vi "Selection.Convert.Set.vi"(8 "error in (no error)":errorcluster, 10 "Selections":T1={"Pull In Time"=FALSE, "Pull In Max Current"=FALSE, "Pull In Max Voltage"=TRUE, "Pull In Min Voltage"=TRUE, "Pull In Avg Voltage"=FALSE, "Hold Time"=FALSE, "Hold Max Current"=FALSE, "Hold Min Current"=FALSE, "Hold Avg Current"=FALSE, "Hold Max Voltage"=FALSE, "Hold Min Voltage"=FALSE, "Hold Avg Max Voltage"=FALSE, "Hold Avg Min Voltage"=FALSE, "Off Time"=FALSE, "Off Max Current"=FALSE, "Off Min Current"=FALSE, "Off Avg Current"=FALSE, "Off Max Voltage"=FALSE, "Off Min Voltage"=TRUE, "Off Avg Voltage"=FALSE, "Total Voltage Pulses"=FALSE, "Total Stage Time"=TRUE}, 11 "ListBox in":refnum<vi>) -> (0 "error out":errorcluster)   [LabVIEW 2019, in "Fuel Injector Analysis Addon System Explorer.lvlib"]
uses:
  Fuel Injector Analysis Addon System Explorer.lvlib
  Addon Shared/Types/Analysis.Channels.Select.ctl
  Addon Shared/Fuel Injector Analysis Addon Shared.lvlib
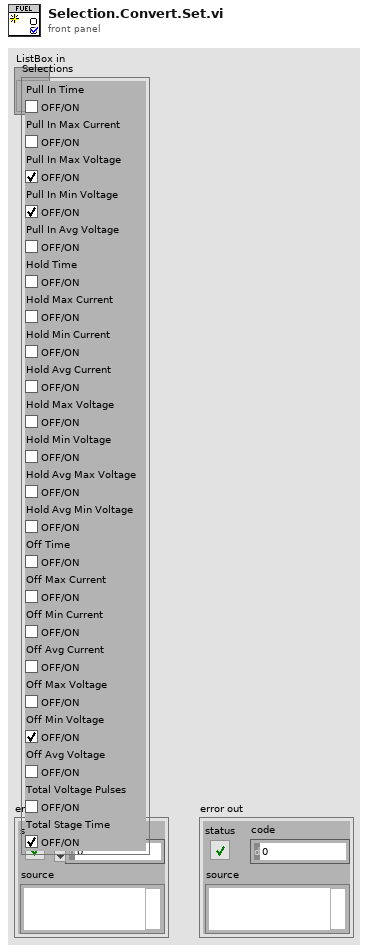
[diagram p1: front panel]
types:
  T1 = typedef "Fuel Injector Analysis Addon Shared.lvlib/Analysis.Channels.Select.ctl" = cluster{"Pull In Time":bool, "Pull In Max Current":bool, "Pull In Max Voltage":bool, "Pull In Min Voltage":bool, "Pull In Avg Voltage":bool, "Hold Time":bool, "Hold Max Current":bool, "Hold Min Current":bool, "Hold Avg Current":bool, "Hold Max Voltage":bool, "Hold Min Voltage":bool, "Hold Avg Max Voltage":bool, "Hold Avg Min Voltage":bool, "Off Time":bool, "Off Max Current":bool, "Off Min Current":bool, "Off Avg Current":bool, "Off Max Voltage":bool, "Off Min Voltage":bool, "Off Avg Voltage":bool, "Total Voltage Pulses":bool, "Total Stage Time":bool}
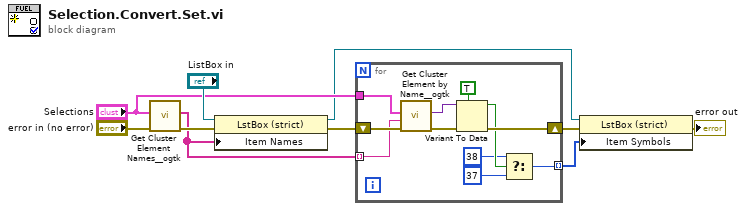
[diagram p0: block diagram]
diagram:
  n1 = call <userlib>:"Get Cluster Element Names__ogtk.vi"("error in (no error)"="error in (no error)", "Cluster"="Selections") -> ("error out"=w6:errorcluster, "Element Names"=w2:string[])  [unwired: 8 in]
  n2 = property class="LstBox (strict)"(reference="ListBox in", error in=w6, "Item Names"=w2) -> (reference out=w5:refnum<vi>, error out=w4:errorcluster)
  n3 = for {
    shift-right: [w16] -> w3
    shift-left: w4 -> [w21]
    tunnel: "Selections" -> [w20]
    tunnel: w2 -> [w19] mode=indexing
    tunnel: [w11] -> w1 mode=indexing
    n4 = call <userlib>:"Get Cluster Element by Name__ogtk.vi"("error in (no error)"=w21, "Element Name"=w19, "Cluster"=w20) -> ("error out"=w18:errorcluster, "VElement"=w17:variant)  [unwired: 6 in, 1 out]
    n5 = Variant To Data(error in=w18, type=TRUE, Variant=w17) -> (data=w14:bool, error out=w16:errorcluster)
    n6 = Select(t=38, s=w14, f=37) -> (s? t:f=w11:i32)
  }
  n7 = property class="LstBox (strict)"(reference=w5, error in=w3, "Item Symbols"=w1) -> (error out=→"error out":errorcluster)  [unwired: 1 out]
